vi "Read ID.vi"(8 "error in (no error)":errorcluster, 11 "Handle":u32) -> (0 "error out":errorcluster, 2 "Data":string, 3 "Status":i32)   [LabVIEW 2016, in "Photon Counter.lvlib" / "C8855-01.lvlib"]
doc: "Returns the ID switch value of this unit.\n\n\nBOOL C8855API __stdcall C8855ReadId( HANDLE hC8855, \n BYTE *Data );"
uses:
  C8855-01.lvlib
  C8855-01api.dll
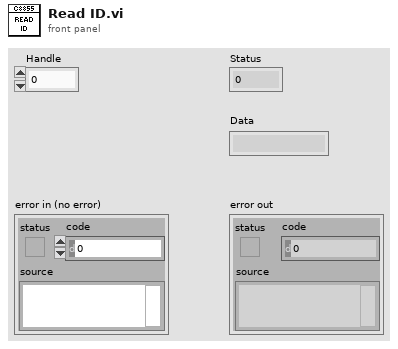
[diagram p1: front panel]
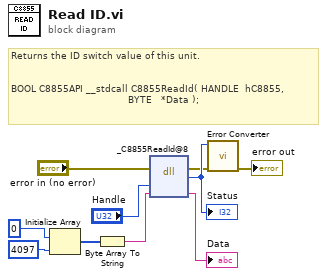
[diagram p0: block diagram]
diagram:
  # "Returns the ID switch value of this unit.\n\n\nBOOL C8855API __stdcall C8855ReadId( HANDLE  hC8855,\t\n                                       BYTE   *Data );"
  n1 = Initialize Array(u8 0 ("element"), 4097 ("dimension size")) -> (w8:u8[])
  n2 = Byte Array To String(unsigned byte array=w8) -> (string=w7:string)
  n3 = dll-call lib="C:/Users/Andy/Desktop/Trace Grabber/Drivers/C8855-01/C8855-01api.*" fn="_C8855ReadId@8"(error in="error in (no error)", "Handle"="Handle", "Data"=w7) -> (error out=w2:errorcluster, w10:i32, "Data"=→"Data":string)  [unwired: 3 in, 1 out]
  "Status" <- w10
  n4 = call "Error Converter.vi"("error in (no error)"=w2, "error code"=w10) -> ("error out"=→"error out":errorcluster)  [unwired: 9 in]
